vi "MediaCH.vi"(0 "input cluster":T1, 7 "nº mitjana":dbl, 11 "I":dbl, 13 "Data":waveform(dbl)[](array[waveform])) -> (4 "Mitja CH1":dbl format="%0.2f", 6 "Mitja CH2":dbl format="%0.2f", 8 "Mitja CH3":dbl format="%0.2f", 10 "Mitja CH4":dbl format="%0.2f")   [LabVIEW 2014]
uses:
  <vilib>/Analysis/baseanly.llb/Mean (DBL).vi
  <vilib>/Waveform/WDTOps.llb/WDT Index Channel DBL.vi
  <vilib>/Analysis/NI_AALBase.lvlib
panel:
  out "subarray":waveform(dbl)[](array[waveform])
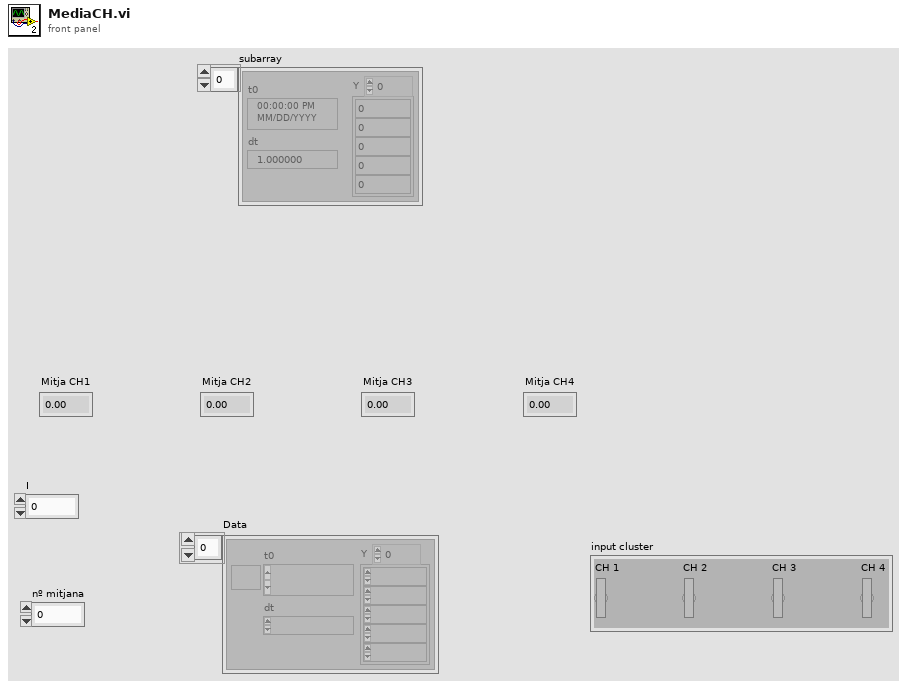
[diagram p1: front panel]
types:
  T1 = cluster{"CH 1":bool, "CH 2":bool, "CH 3":bool, "CH 4":bool}
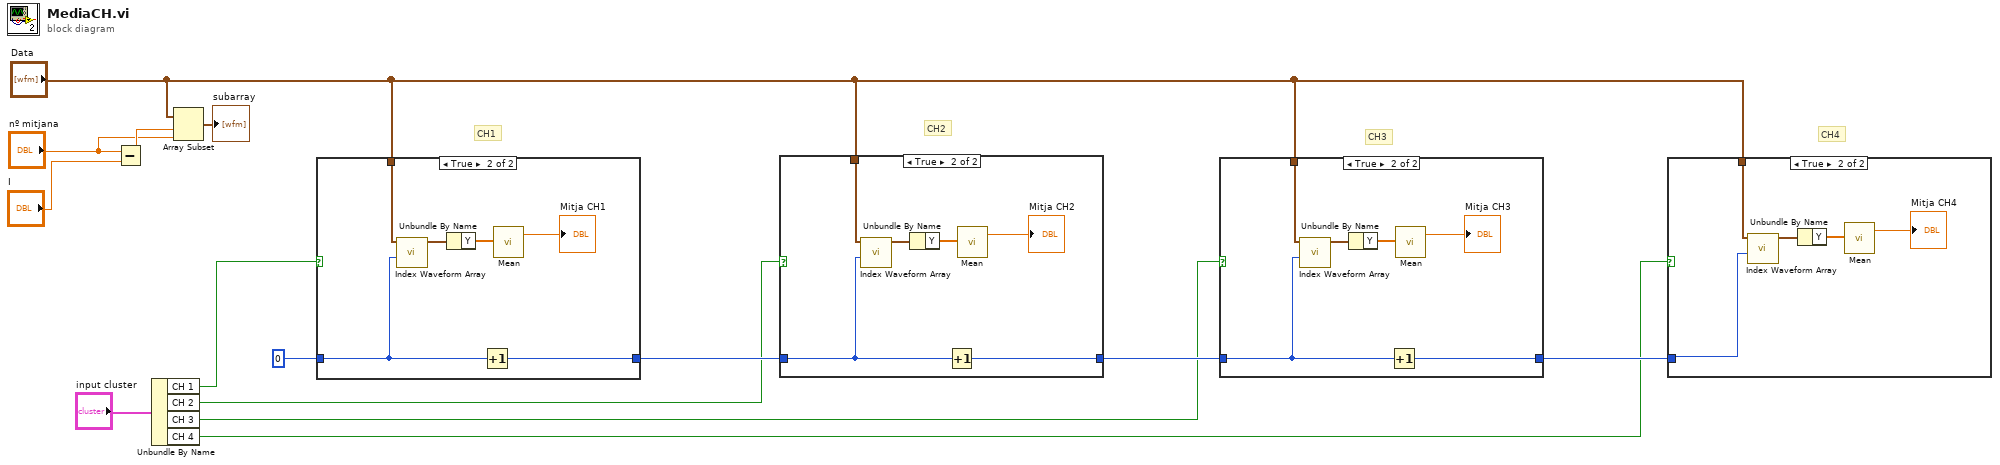
[diagram p0: block diagram]
diagram:
  # "CH4"
  # "CH3"
  # "CH2"
  # "CH1"
  n1 = Subtract(x="nº mitjana", y="I") -> (x-y=w4:dbl)
  n2 = Unbundle By Name("input cluster") -> ("CH 1"=w9:bool, "CH 2"=w8:bool, "CH 3"=w7:bool, "CH 4"=w6:bool)
  n3 = Array Subset(array="Data", index=w4, length="nº mitjana") -> (→"subarray":waveform(dbl)[])
  n4 = case shown="True" w9 {
    tunnel: 0 -> [w15 w19]
    tunnel: [w15 w17] -> w13
    tunnel: "Data" -> [_ w16]
    frame False {
    }
    frame True {
      n5 = call-poly <vilib>:"Index Waveform Array.vi"("index"=w19, "waveform array"=w16) -> ("waveform"=w18:waveform(dbl))  [unwired: 8 in, 1 out]
      n6 = Unbundle By Name(w18) -> ("Y"=w21:dbl[])
      n7 = Increment(x=w19) -> (x+1=w17:i32)
      n8 = call-poly <vilib>:"Mean.vi"("X"=w21) -> ("mean"=→"Mitja CH1":dbl)  [unwired: 1 out]
    }
  }
  n9 = case shown="True" w8 {
    tunnel: w13 -> [w22 w25]
    tunnel: [w22 w24] -> w12
    tunnel: "Data" -> [_ w23]
    frame False {
    }
    frame True {
      n10 = call-poly <vilib>:"Index Waveform Array.vi"("index"=w25, "waveform array"=w23) -> ("waveform"=w28:waveform(dbl))  [unwired: 8 in, 1 out]
      n11 = Unbundle By Name(w28) -> ("Y"=w27:dbl[])
      n12 = Increment(x=w25) -> (x+1=w24:i32)
      n13 = call-poly <vilib>:"Mean.vi"("X"=w27) -> ("mean"=→"Mitja CH2":dbl)  [unwired: 1 out]
    }
  }
  n14 = case shown="True" w7 {
    tunnel: w12 -> [w29 w32]
    tunnel: [w29 w31] -> w11
    tunnel: "Data" -> [_ w30]
    frame False {
    }
    frame True {
      n15 = call-poly <vilib>:"Index Waveform Array.vi"("index"=w32, "waveform array"=w30) -> ("waveform"=w35:waveform(dbl))  [unwired: 8 in, 1 out]
      n16 = Unbundle By Name(w35) -> ("Y"=w34:dbl[])
      n17 = Increment(x=w32) -> (x+1=w31:i32)
      n18 = call-poly <vilib>:"Mean.vi"("X"=w34) -> ("mean"=→"Mitja CH3":dbl)  [unwired: 1 out]
    }
  }
  n19 = case shown="True" w6 {
    tunnel: w11 -> [_ w37]
    tunnel: "Data" -> [_ w36]
    frame False {
    }
    frame True {
      n20 = call-poly <vilib>:"Index Waveform Array.vi"("index"=w37, "waveform array"=w36) -> ("waveform"=w40:waveform(dbl))  [unwired: 8 in, 1 out]
      n21 = Unbundle By Name(w40) -> ("Y"=w39:dbl[])
      n22 = call-poly <vilib>:"Mean.vi"("X"=w39) -> ("mean"=→"Mitja CH4":dbl)  [unwired: 1 out]
    }
  }
